vi "lm35_sukur.vi"() -> ()   [LabVIEW 2017]
uses:
  <vilib>/MakerHub/LINX/Public/Peripherals/Analog/Analog Read 1 Chan.vi
  <vilib>/MakerHub/LINX/Public/Peripherals/Analog/Analog Read N Chans.vi
  <vilib>/MakerHub/LINX/Private/Local IO/LinxAnalogRead.vi
  <vilib>/MakerHub/LINX/Public/Utilities/Check Channel.vi
  <vilib>/MakerHub/LINX/Public/Utilities/Open Serial.vi
  <vilib>/MakerHub/LINX/Private/Utilties/Generate Error.vi
  <vilib>/Utility/NIReport.llb/Append Report Text (str wrap).vi
  <vilib>/printing/ReportDocExtensions.llb/Append Front Panel Image to Report (path).vi
  <vilib>/Utility/NIReport.llb/NI_report.lvclass
  <vilib>/MakerHub/LINX/LMH-LINX.lvlib
  <vilib>/Utility/NIReport.llb/NI_ReportGenerationCore.lvlib
panel:
  out "Numeric":dbl
  in  "stop":bool
  out "Thermometer":dbl(slide) scale=0.0..100.0
  in  "Analog Channel":u8
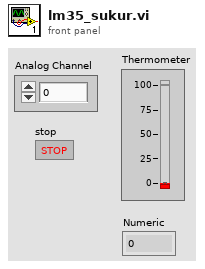
[diagram p1: front panel]
types:
  T1 = cluster{"top":dbl, "left":dbl, "right":dbl, "bottom":dbl}
  T2 = cluster{"Charset (-1)":i16, "Weight (-1)":i16, "Name":string, "Size":string}
  T3 = cluster{"Italic":enum16{"Italic Unchanged", "Italic On", "Italic Off"}, "Strike Through":enum16{"Strike Through Unchanged", "Strike Through On", "Strike Through Off"}, "Underline":enum16{"Underline Unchanged", "Underline On", "Underline Off"}, "Bold":enum16{"Bold Unchanged", "Bold On", "Bold Off"}}
  T4 = enum16{"Standard Report", "HTML", "Word", "Excel"}
  T5 = typedef "LMH-LINX.lvlib/LINX Ref.ctl" = cluster{"IO":T6, "Interface":T7, "LINX Device Config":T8}
  T6 = typedef "LMH-LINX.lvlib/Platform.ctl" = enum16{"Remote", "Local"}
  T7 = typedef "LMH-LINX.lvlib/Interface.ctl" = enum16{"Serial", "TCP"}
  T8 = typedef "LMH-LINX.lvlib/Device.lvlib/LINX Device Config.ctl" = cluster{"Interface":T7, "COM Port":refnum<visa-resource-name>, "TCP Configuration":T9, "Device Family":u8, "Device ID":u8, "Device Name":string, "TCP Ref":refnum<k5>, "Channels":T10}
  T9 = typedef "LMH-LINX.lvlib/Device.lvlib/TCP Config.ctl" = cluster{"IP Address":string, "Port":u16}
  T10 = typedef "LMH-LINX.lvlib/Channels.ctl" = cluster{"DI":u8[], "DO":u8[], "AI":u8[], "AO":u8[], "PWM":u8[], "QE":u8[], "UART":u8[], "I2C 2":u8[], "SPI":u8[], "CAN":u8[], "Servo":u8[], "AI Ref (V)":dbl, "AI Resolution (Bits)":u8, "AO Ref (V)":dbl, "AO Resolution (Bits)":u8}
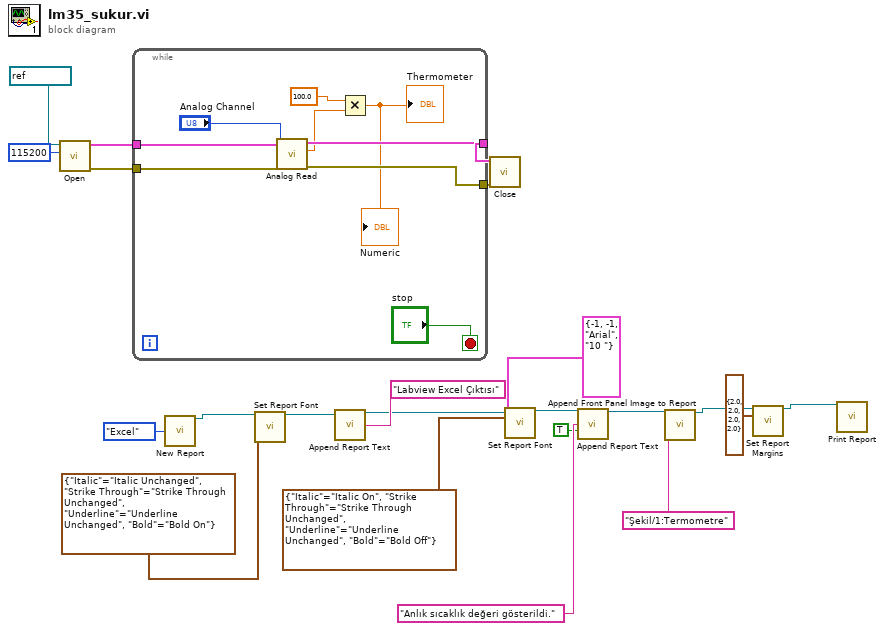
[diagram p0: block diagram]
diagram:
  n1 = call-poly <vilib>:"Open.vi"("Baud Rate Override"=u32 115200, "Serial Port"=refnum<visa-resource-name> "COM4") -> ("Error Out"=w18:errorcluster, "LINX Resource"=w20:T5)  [unwired: 7 in, 1 out]
  n2 = while {
    tunnel: w20 -> [w31]
    tunnel: [w30] -> w19
    tunnel: w18 -> [w29]
    tunnel: [w28] -> w17
    stop <- "stop" stop-if-true
    n3 = call-poly <vilib>:"Analog Read.vi"("Error In"=w29, "Analog Channel"="Analog Channel", "LINX Resource"=w31) -> ("Error Out"=w28:errorcluster, "Voltage"=w26:dbl, "LINX Resource"=w30:T5)  [unwired: 5 in, 1 out]
    n4 = Multiply(x=100.0, y=w26) -> (x*y=→"Thermometer" →"Numeric":dbl)
  }
  n5 = call <vilib>:"New Report.vi"("report type"=T4."Excel") -> ("report out"=w16:refnum<class "NI_report.lvclass">)  [unwired: 13 in, 1 out]
  n6 = call-dynamic "Set Report Font.vi"("report in"=w16, "text options"=T3 {"Italic"=enum."Italic Unchanged", "Strike Through"=enum."Strike Through Unchanged", "Underline"=enum."Underline Unchanged", "Bold"=enum."Bold On"}) -> ("report out"=w12:refnum<class "NI_report.lvclass">)  [unwired: 11 in, 2 out]
  n7 = call-poly <vilib>:"Append Report Text.vi"("report in"=w12, "text"="Labview Excel Çıktısı") -> ("report out"=w11:refnum<class "NI_report.lvclass">)  [unwired: 10 in, 3 out]
  n8 = call <vilib>:"Close.vi"("Error In"=w17, "LINX Resource"=w19) -> ()  [unwired: 9 in, 1 out]
  n9 = call-dynamic "Set Report Font.vi"("report in"=w11, "text options"=T3 {"Italic"=enum."Italic On", "Strike Through"=enum."Strike Through Unchanged", "Underline"=enum."Underline Unchanged", "Bold"=enum."Bold Off"}, "font settings"=T2 {"Charset (-1)"=-1, "Weight (-1)"=-1, "Name"="Arial", "Size"="10 "}) -> ("report out"=w8:refnum<class "NI_report.lvclass">)  [unwired: 10 in, 2 out]
  n10 = call-poly <vilib>:"Append Report Text.vi"("report in"=w8, "text"="Anlık sıcaklık değeri gösterildi.", "append on new line? (F)"=TRUE) -> ("report out"=w6:refnum<class "NI_report.lvclass">)  [unwired: 9 in, 3 out]
  n11 = call-poly <vilib>:"Append Front Panel Image to Report.vi"("report in"=w6, "description"="Şekil/1:Termometre") -> ("report out"=w4:refnum<class "NI_report.lvclass">)  [unwired: 9 in, 4 out]
  n12 = call-dynamic "Set Report Margins.vi"("report in"=w4, "margins (1.00)"=T1 {"top"=2.0, "left"=2.0, "right"=2.0, "bottom"=2.0}) -> ("report out"=w2:refnum<class "NI_report.lvclass">)  [unwired: 11 in, 2 out]
  n13 = call-dynamic "Print Report.vi"("report in"=w2) -> ()  [unwired: 13 in, 2 out]
